vi "TakeLaserlessImage.vi"(8 "error in":errorcluster, 10 "Image In":T2, 11 "Session In":T1) -> (0 "error out":errorcluster, 2 "nolaser Filepath":path, 3 "Session Out":T1)   [LabVIEW 2014]
uses:
  <vilib>/userdefined/High Color/IMAQdx.ctl
  <vilib>/vision/Image Controls.llb/IMAQ Image.ctl
  <vilib>/vision/driver/NI_Vision_Acquisition_Software.lvlib
panel:
  in  "Take Picture":bool
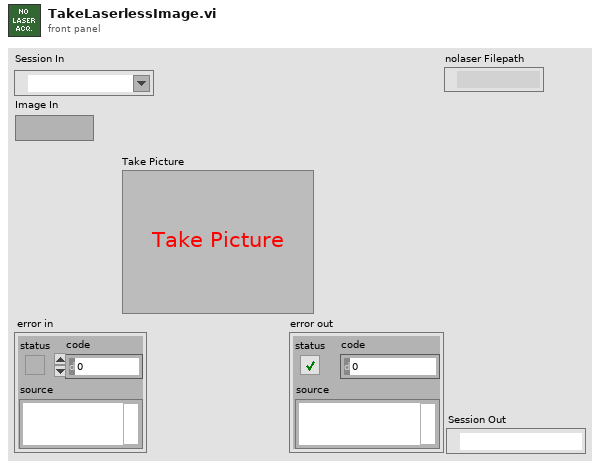
[diagram p1: front panel]
types:
  T1 = typedef "IMAQdx.ctl" = refnum<k21>
  T2 = typedef "IMAQ Image.ctl" = refnum<image>
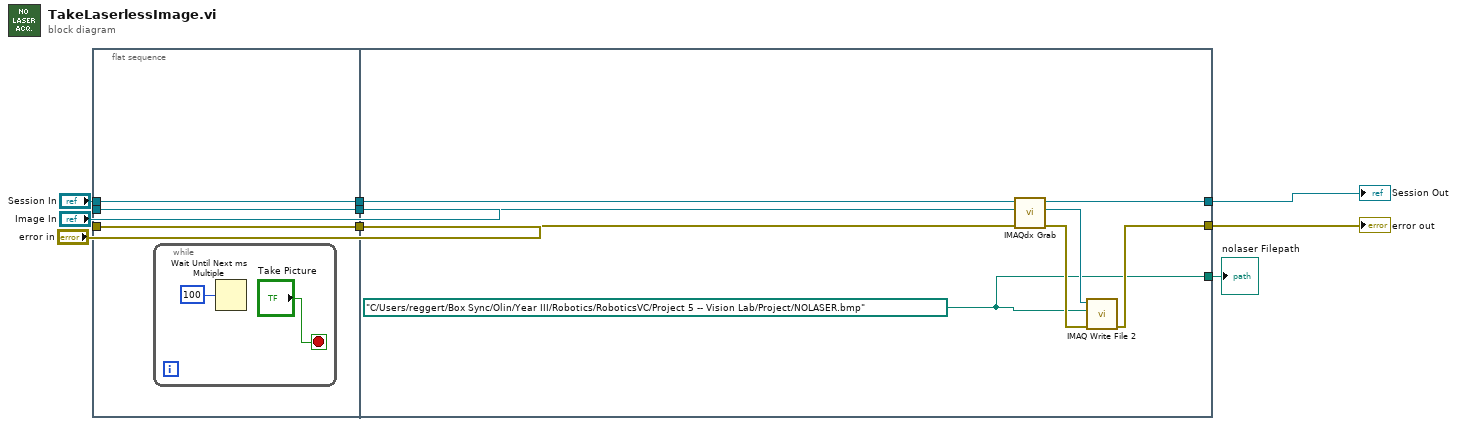
[diagram p0: block diagram]
diagram:
  n1 = flat-sequence {
    tunnel: "Session In" -> [w12]
    tunnel: [w12] -> w9
    tunnel: "Image In" -> [w11]
    tunnel: [w11] -> w6
    tunnel: [w10] -> w5
    tunnel: "error in" -> [w10]
    tunnel: [w16] -> w3
    tunnel: [w22] -> w2
    tunnel: w9 -> [w21]
    tunnel: w6 -> [w20]
    tunnel: w5 -> [w19]
    tunnel: [w15] -> w1
    frame #0 {
      n2 = while {
        stop <- "Take Picture" stop-if-true
        n3 = Wait Until Next ms Multiple(millisecond multiple=u32 100 ("milliseconds to wait")) -> ()  [unwired: 1 out]
      }
    }
    frame #1 {
      w15 = path "C:/Users/reggert/Box Sync/Olin/Year III/Robotics/RoboticsVC/Project 5 -- Vision Lab/Project/NOLASER.bmp" ("File Path")
      n4 = call <vilib>:"IMAQdx Grab.vi"("error in"=w19, "Image In"=w20, "Session In"=w21) -> ("error out"=w17:errorcluster, "Image Out"=w18:T2, "Session Out"=w22:T1)  [unwired: 1 in, 5 out]
      n5 = call-poly "IMAQ Write File 2"("error in (no error)"=w17, "File Path"=w15, "Image"=w18) -> ("error out"=w16:errorcluster)  [unwired: 7 in, 1 out]
    }
  }
  "error out" <- w3
  "Session Out" <- w2
  "nolaser Filepath" <- w1
